vi "Test Build Library HTML Documentation.vi"   [LabVIEW 2018, in "Scripts.lvlib"]
uses:
  Scripts.lvlib
  <vilib>/Field R&D Services/Labricator/Toolkit/Labricator.lvlib
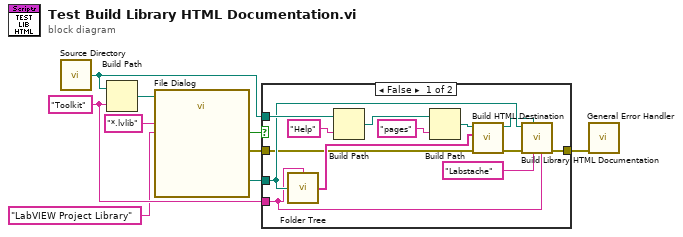
[diagram p0: block diagram]
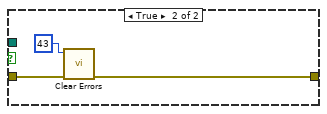
[diagram p2: hidden frame]
diagram:
  w4 = "Toolkit" ("Root Folder Name")
  n1 = call <vilib>:"Source Directory.vi"() -> ("Source Directory"=w5:path)
  n2 = Build Path(base path=w5, name or relative path=w4) -> (appended path=w3:path)
  n3 = call "File Dialog"("start path"=w3, "pattern (all files)"="*.lvlib", "pattern label"="LabVIEW Project Library") -> ("selected path"=w6:path, "cancelled"=w9:bool, "error out"=w8:errorcluster)  [unwired: 9 in, 1 out]
  n4 = case shown="False" w9 {
    tunnel: w8 -> [w14 w25]
    tunnel: [w22 w23] -> w7
    tunnel: w6 -> [w15 _]
    tunnel: w5 -> [w19 _]
    tunnel: w4 -> [w10 _]
    frame False {
      n5 = call "Folder Tree.vi"("File"=w15, "Root Folder Name"=w10) -> ("Hierarchy Folders"=w16:string[])
      n6 = Build Path(base path=w19, name or relative path="Help") -> (appended path=w18:path)
      n7 = Build Path(base path=w18, name or relative path="pages") -> (appended path=w11:path)
      n8 = call "Build HTML Destination.vi"("Error In"=w14, "Hierarchy Folders"=w16, "Root Destination"=w11) -> ("Error Out"=w13:errorcluster, "HTML Destination"=w12:path)  [unwired: 7 in]
      n9 = call "Build Library HTML Documentation.vi"("Root Folder Name"=w10, "Requirement"="Labstache", "Destination"=w12, "Error In"=w13, "Library File"=w15) -> ("Error Out"=w22:errorcluster)  [unwired: 6 in]
    }
    frame True {
      n10 = call <vilib>:"Clear Errors.vi"("error in (no error)"=w25, "specific error code to clear (0: all)"=43) -> ("error out"=w23:errorcluster)  [unwired: 4 in, 1 out]
    }
  }
  n11 = call <vilib>:"General Error Handler.vi"("error in (no error)"=w7) -> ()  [unwired: 10 in, 5 out]
